vi "createCommand.vi"(8 "error in (no error)":errorcluster, 9 "Variant":variant, 10 "Command":T1, 11 "SpectrographClientCommunicator in":refnum<class "SpectrographClientCommunicator.lvclass">) -> (0 "error out":errorcluster, 2 "command":string, 3 "SpectrographClientCommunicator out":refnum<class "SpectrographClientCommunicator.lvclass">)   [LabVIEW 2016, in "SpectrographClientCommunicator.lvclass"]
uses:
  SpectrographClientCommunicator.lvclass
  SpectrographTypeDef/SpectrographCMDs.ctl
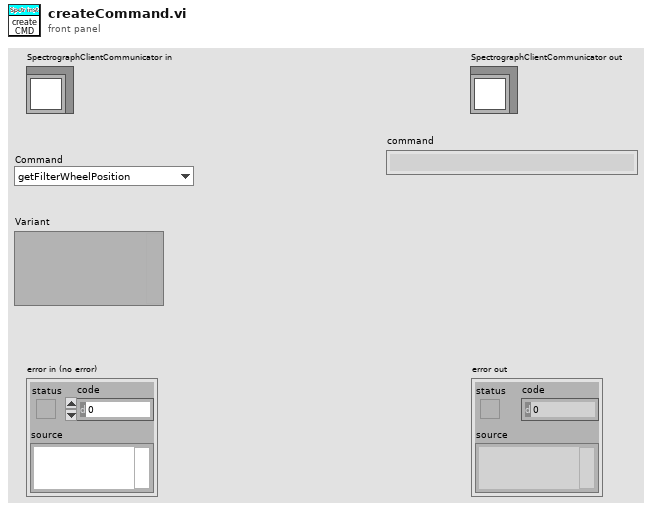
[diagram p1: front panel]
types:
  T1 = typedef "SpectrographCMDs.ctl" = enum16{"getFilterWheelPosition", "getGratingWheelPosition", "moveLinearStage", "moveGratingWheel", "moveFilterWheel", "homeLinearStage", "getLinearStageStatus", "getGratingWheelStatus", "getFilterWheelStatus", "stopAllMotion"}
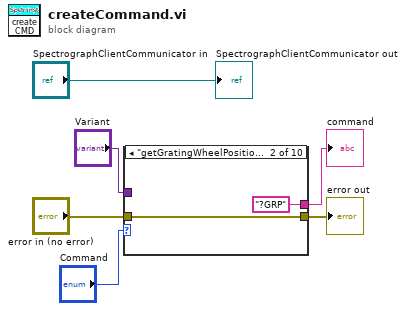
[diagram p0: block diagram]
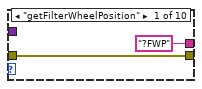
[diagram p2: hidden frame]
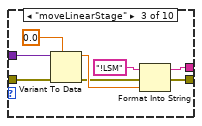
[diagram p3: hidden frame]
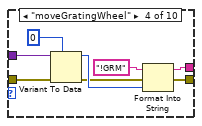
[diagram p4: hidden frame]
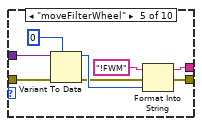
[diagram p5: hidden frame]
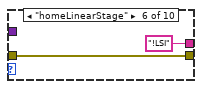
[diagram p6: hidden frame]
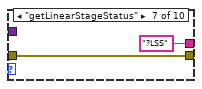
[diagram p7: hidden frame]
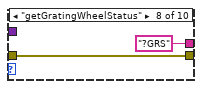
[diagram p8: hidden frame]
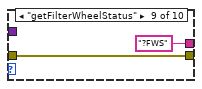
[diagram p9: hidden frame]
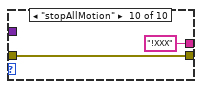
[diagram p10: hidden frame]
diagram:
  n1 = case shown="\"getGratingWheelPosition\"" "Command" {
    tunnel: "Variant" -> [_ _ w16 w22 w29 _ _ _ _ _]
    tunnel: ["?FWP" "?GRP" w13 w20 w28 "!LSI" "?LSS" "?GRS" "?FWS" "!XXX"] -> w3
    tunnel: "error in (no error)" -> [w7 w9 w18 w23 w30 w35 w37 w39 w42 w44]
    tunnel: [w7 w9 w11 w19 w27 w35 w37 w39 w42 w44] -> w1
    frame "getFilterWheelPosition" {
    }
    frame "getGratingWheelPosition" {
    }
    frame "moveLinearStage" {
      n2 = Variant To Data(error in=w18, type=0.0 ("Linear Stage Position"), Variant=w16) -> (data=w14:dbl, error out=w12:errorcluster)
      n3 = Format Into String(initial string="!LSM", error in=w12, w14) -> (resulting string=w13:string, error out=w11:errorcluster)  [unwired: 1 in]
    }
    frame "moveGratingWheel" {
      n4 = Variant To Data(error in=w23, type=u8 0 ("Grating Wheel Position"), Variant=w22) -> (data=w25:u8, error out=w24:errorcluster)
      n5 = Format Into String(initial string="!GRM", error in=w24, w25) -> (resulting string=w20:string, error out=w19:errorcluster)  [unwired: 1 in]
    }
    frame "moveFilterWheel" {
      n6 = Variant To Data(error in=w30, type=u8 0 ("Grating Wheel Position"), Variant=w29) -> (data=w33:u8, error out=w32:errorcluster)
      n7 = Format Into String(initial string="!FWM", error in=w32, w33) -> (resulting string=w28:string, error out=w27:errorcluster)  [unwired: 1 in]
    }
    frame "homeLinearStage" {
    }
    frame "getLinearStageStatus" {
    }
    frame "getGratingWheelStatus" {
    }
    frame "getFilterWheelStatus" {
    }
    frame "stopAllMotion" {
    }
  }
  "error out" <- w1
  "command" <- w3
  "SpectrographClientCommunicator out" <- "SpectrographClientCommunicator in"
